vi "GetAttributeViInt32_ACP_SE_TOI.vi"(8 "error in (no error)":errorcluster {"code" format="%.0x"}, 9 "AttributeID":u32(ring)=1150128 items=["SA_ACP_AVERAGE_COUNT"=1150128, "SA_ACP_AVERAGE_MODE"=1150130, "SA_ACP_CARRIER_COUNT"=1150138, "SA_ACP_CARRIER_REFERENCE_NUMBER"=1150144, "SA_ACP_DETECTOR_TYPE"=1150123, "SA_ACP_DISPLAY_WINDOWY_REF_POSITION"=1150149, "SA_ACP_FREQUENCY_PHASE_NOISE_OPTION_STATE"=1150153, "SA_ACP_MARKER_ACTIVE_MARKER"=1150233, "SA_ACP_MARKER_COUNT"=1150235, "SA_ACP_MARKER_DELTA_REFERENCE"=1150237, "SA_ACP_MARKER_TRACE"=1150241, "SA_ACP_MARKER_TYPE"=1150242, "SA_ACP_MEASUREMENT_METHOD"=1150125, "SA_ACP_MEASUREMENT_TYPE"=1150126, "SA_ACP_OFFSET_TYPE"=1150419, "SA_ACP_SWEEPCOUPLING_BANDWIDTH_SHAPE"=1150134, "SA_ACP_SWEEPCOUPLING_BANDWIDTH_TYPE"=1150135, "SA_ACP_SWEEPCOUPLING_SWEEP_POINTS"=1150167, "SA_ACP_SWEEPCOUPLING_SWEEP_TIME_AUTO_RULES"=1150170, "SA_ACP_TRACE_TYPE"=1150776, "SA_ACP_TRIGGER_SOURCE"=1150127, "SA_SPURIOUS_EMISSION_DISPLAY_VIEW_SELECTION "=1150821, "SA_SPURIOUSEMISSIONS_AVERAGE_COUNT"=1150423, "SA_SPURIOUSEMISSIONS_AVERAGE_MODE"=1150425, "SA_SPURIOUSEMISSIONS_DISPLAY_VIEW"=1150453, "SA_SPURIOUSEMISSIONS_MARKER_ACTIVE_MARKER"=1150438, "SA_SPURIOUSEMISSIONS_MARKER_COUNT"=1150440, "SA_SPURIOUSEMISSIONS_MARKER_DELTA_REFERENCE"=1150442, "SA_SPURIOUSEMISSIONS_MARKER_TRACE"=1150446, "SA_SPURIOUSEMISSIONS_MARKER_TYPE"=1150447, "SA_SPURIOUSEMISSIONS_MEASUREMENT_TYPE"=1150428, "SA_SPURIOUSEMISSIONS_REPORT_MODE"=1150429, "SA_SPURIOUSEMISSIONS_TRIGGER_SOURCE"=1150430, "SA_THIRDORDERINTERCEPT_AVERAGE_COUNT"=1150482, "SA_THIRDORDERINTERCEPT_AVERAGE_MODE"=1150484, "SA_THIRDORDERINTERCEPT_DISPLAYWINDOWY_REF_POSITION"=1150580, "SA_THIRDORDERINTERCEPT_SWEEPCOUPLING_SWEEP_POINTS"=1150488, "SA_THIRDORDERINTERCEPT_TRACES_TYPE"=1150781, "SA_THIRDORDERINTERCEPT_TRIGGER_SOURCE"=1150495], 10 "RepCapIdentifier":string, 11 "instrument handle":refnum<k15>) -> (0 "error out":errorcluster {"code" format="%.0x"}, 2 "AttributeValue":i32, 3 "instrument handle out":refnum<k15>)   [LabVIEW 2009, in "Keysight XSAn.lvlib"]
doc: "Gets an Int32 attribute from the instrument driver.\nThe following Attributes are supported:\n\nSA_ACP_AVERAGE_COUNT\nSA_ACP_AVERAGE_MODE\nSA_ACP_CARRIER_COUNT\nSA_ACP_CARRIER_REFERENCE_NUMBER\nSA_ACP_DETECTOR_TYPE\nSA_ACP_DISPLAY_WINDOWY_REF_POSITION\nSA_ACP_FREQUENCY_PHASE_NOISE_OPTION_STATE\nSA_ACP_MARKER_ACTIVE_MARKER\nSA_ACP_MARKER_COUNT\nSA_ACP_MARKER_DELTA_REFERENCE\nSA_ACP_MARKER_TRACE\nSA_ACP_MARKER_TYPE\nSA_ACP_MEASUREMENT_METHOD\nSA_ACP_MEASUREMENT_TYPE\nSA_ACP_OFFSET_TYPE\nSA_ACP_SWEEPCOUPLING_BANDWIDTH_SHAPE\nSA_ACP_SWEEPCOUPLING_BANDWIDTH_TYPE\nSA_ACP_SWEEPCOUPLING_SWEEP_POINTS\nSA_ACP_SWEEPCOUPLING_SWEEP_TIME_AUTO_RULES\nSA_ACP_TRACE_TYPE\nSA_ACP_TRIGGER_SOURCE\nSA_SPURIOUS_EMISSION_DISPLAY_VIEW_SELECTION \nSA_SPURIOUSEMISSIONS_AVERAGE_COUNT\nSA_SPURIOUSEMISSIONS_AVERAGE_MODE\nSA_SPURIOUSEMISSIONS_DISPLAY_VIEW\nSA_SPURIOUSEMISSIONS_MARKER_ACTIVE_MARKER\nSA_SPURIOUSEMISSIONS_MARKER_COUNT\nSA_SPURIOUSEMISSIONS_MARKER_DELTA_REFERENCE\nSA_SPURIOUSEMISSIONS_MARKER_TRACE\nSA_SPURIOUSEMISSIONS_MARKER_TYPE\nSA_SPURIOUSEMISSIONS_MEASUREMENT_TYPE\nSA_SPURIOUSEMISSIONS_REPORT_MODE\nSA_SPURIOUSEMISSIONS_TRIGGER_SOURCE\nSA_THIRDORDERINTERCEPT_AVERAGE_COUNT\nSA_THIRDORDERINTERCEPT_AVERAGE_MODE\nSA_THIRDORDERINTERCEPT_DISPLAYWINDOWY_REF_POSITION\nSA_THIRDORDERINTERCEPT_SWEEPCOUPLING_SWEEP_POINTS\nSA_THIRDORDERINTERCEPT_TRACES_TYPE\nSA_THIRDORDERINTERCEPT_TRIGGER_SOURCE"
uses:
  <instrlib>/Keysight XSAn/Keysight XSAn.lvlib
  AgXSAn.dll
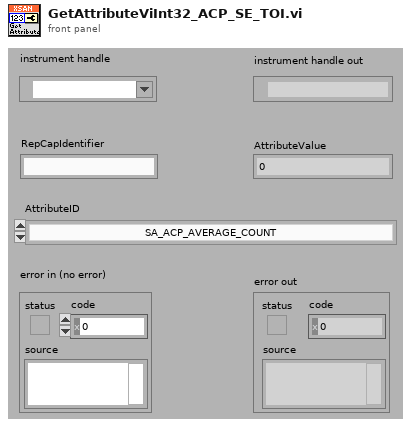
[diagram p1: front panel]
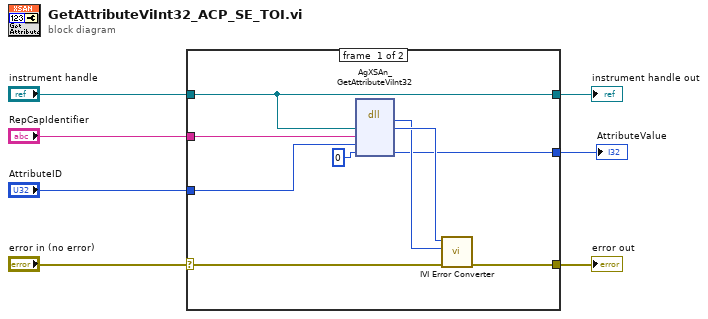
[diagram p0: block diagram]
diagram:
  n1 = case shown="No Error" "error in (no error)" {
    selector: "error in (no error)" -> [w14 w18]
    tunnel: [w13 w18] -> w7
    tunnel: "instrument handle" -> [w9 w17]
    tunnel: "AttributeID" -> [w12 _]
    tunnel: [w10 _] -> w3
    tunnel: [w9 w17] -> w2
    tunnel: "RepCapIdentifier" -> [w8 _]
    frame #0 {
      n2 = dll-call lib="AgXSAn**.dll" fn="AgXSAn_GetAttributeViInt32"("Vi"=w9, "RepCapIdentifier"=w8, "AttributeID"=w12, "AttributeValue"=0) -> ("return type"=w15:i32, "Vi"=w16:u32, "AttributeValue"=w10:i32)  [unwired: 5 in, 2 out]
      n3 = call <instrlib>:"IVI Error Converter.vi"("error in (no error)"=w14, "IVI error code (0)"=w15, "instrument handle"=w16) -> ("error out"=w13:errorcluster)  [unwired: 7 in, 1 out]
    }
    frame #1 {
    }
  }
  "error out" <- w7
  "instrument handle out" <- w2
  "AttributeValue" <- w3
